vi "Load From File.vi"(8 "error in (no error)":errorcluster, 10 "Sudoku File":path) -> (0 "error out":errorcluster, 3 "Sudoku String":T1)   [LabVIEW 2015, in "Sudoku Library.lvlib"]
doc: "Created IvanLis by LabVIEW Portal\nProfile: http://labviewportal.org/memberlist.php?mode=viewprofile&u=987\neMail: IvanLisanov@gMail.com\nTelegram: https://t.me/IvanLis"
uses:
  Sudoku Library.lvlib
  TypeDef/Sudoku String.ctl
  <vilib>/Utility/file.llb/Read Delimited Spreadsheet (string).vi
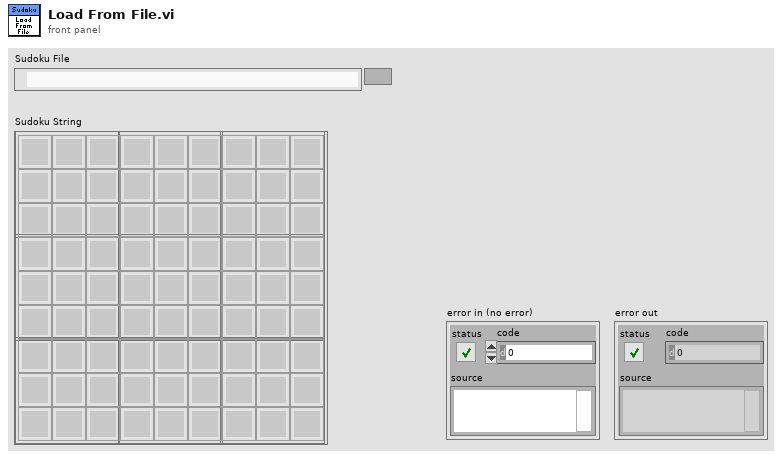
[diagram p1: front panel]
types:
  T1 = typedef "Sudoku Library.lvlib/Sudoku String.ctl" = string[][]
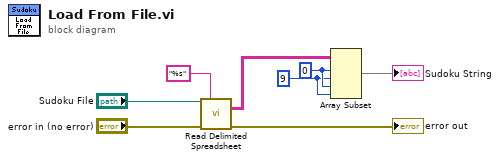
[diagram p0: block diagram]
diagram:
  w1 = 9 ("length")
  w2 = 0 ("index")
  n1 = call-poly <vilib>:"Read Delimited Spreadsheet.vi"("file path (dialog if empty)"="Sudoku File", "format (%s)"="%s" ("format (%.3f)"), "error in (no error)"="error in (no error)") -> ("all rows"=w3:string[][], "error out"=→"error out":errorcluster)  [unwired: 7 in, 4 out]
  n2 = Array Subset(array=w3, index (row)=w2, length (row)=w1, index (col)=w2, length (col)=w1) -> (→"Sudoku String":string[][])
